vi "Read present.vi"(8 "error in (no error)":errorcluster, 11 "Serial IO in":refnum<class "Serial IO.lvclass">) -> (0 "error out":errorcluster, 2 "present?":bool=TRUE, 3 "Serial IO out":refnum<class "Serial IO.lvclass">)   [LabVIEW 2013, in "Serial IO.lvclass"]
uses:
  Serial IO.lvclass
  Serial IO.lvclass/Serial IO.ctl
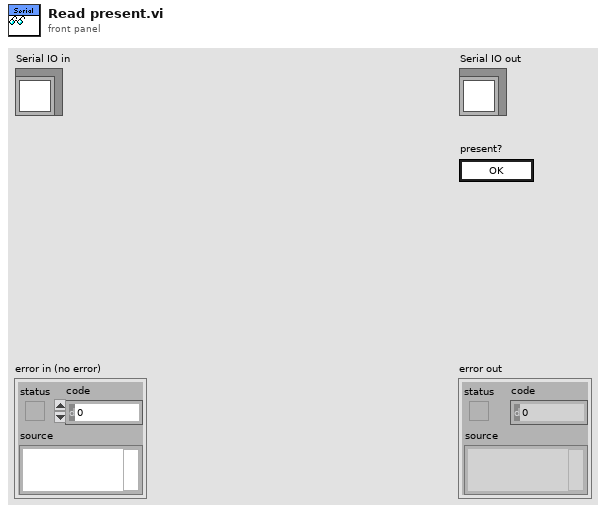
[diagram p1: front panel]
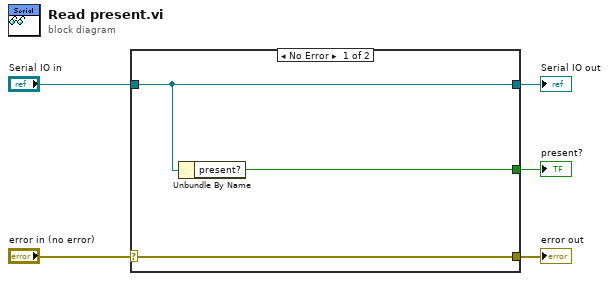
[diagram p0: block diagram]
diagram:
  n1 = case shown="No Error" "error in (no error)" {
    selector: "error in (no error)" -> [w8 w9]
    tunnel: [w8 w9] -> w4
    tunnel: [w7 w10] -> w2
    tunnel: "Serial IO in" -> [w7 w10]
    tunnel: [w6 _] -> w1
    frame No Error {
      n2 = Unbundle By Name(w7) -> ("present?"=w6:bool)
    }
    frame Error {
    }
  }
  "error out" <- w4
  "Serial IO out" <- w2
  "present?" <- w1
